vi "code.vi"(7 "LabVIEW Web Service Request":refnum<class "Web Request.lvclass">) -> ()   [LabVIEW 2015]
uses:
  <vilib>/wsapi/Web Request.lvclass
  lv-dropbox-examples/lv-dropbox-examples.lvlib
  lv-dropbox-examples/private/_controls/authorization_response.ctl
panel:
  # "Use the Web Service Request input terminal to call the VIs on the Web Services palette. Do not remove it from the connector pane unless you don't need access to the palette."
  # "Each additional control wired to the connector pane will be available as an input in the URL. To include an indicator in terminal-mode output (the default setting), it must also be wired to the connector pane."
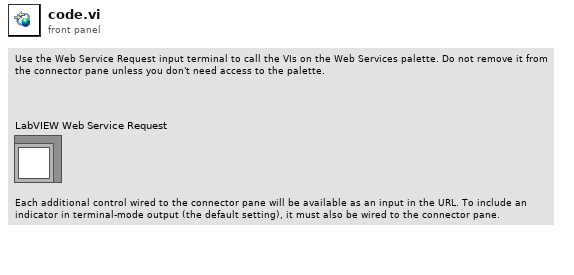
[diagram p1: front panel]
types:
  T1 = typedef "lv-dropbox-examples.lvlib/authorization_response.ctl" = cluster{"code":string, "state":string}
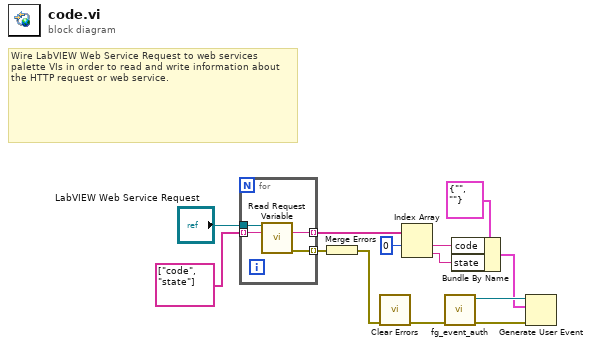
[diagram p0: block diagram]
diagram:
  # "Wire LabVIEW Web Service Request to web services palette VIs in order to read and write information about the HTTP request or web service."
  n1 = for {
    tunnel: "LabVIEW Web Service Request" -> [w17]
    tunnel: string[] ["code", "state"] -> [w16] mode=indexing
    tunnel: [w15] -> w7 mode=indexing
    tunnel: [w14] -> w3 mode=indexing
    n2 = call <vilib>:"Read Request Variable.vi"("LabVIEW Web Service Request"=w17, "variable name"=w16) -> ("value"=w15:string, "error out"=w14:errorcluster)  [unwired: 11 in, 1 out]
  }
  n3 = Merge Errors(w3) -> (w2:errorcluster)
  n4 = call <vilib>:"Clear Errors.vi"("error in (no error)"=w2) -> ("error out"=w1:errorcluster)  [unwired: 5 in, 1 out]
  n5 = Index Array(array=w7, index #1=0 ("index")) -> (element #1=w6:string, element #2=w5:string)  [unwired: 1 in]
  n6 = call "fg_event_auth.vi"("error in (no error)"=w1) -> ("error out"=w10:errorcluster, "auth"=w11:refnum<user-event>)  [unwired: 9 in]
  n7 = Bundle By Name(cluster=T1 {"code"="", "state"=""} ("event data"), "code"=w6, "state"=w5) -> (w8:T1)
  n8 = Generate User Event(user event=w11, event data cluster=w8, error in=w10) -> ()  [unwired: 1 in, 2 out]
